vi "LightFieldParams.vi"(5 "On CCD Accumulations":i32=3 min=0 step=1, 7 "Number of Frames":i32=500 min=0 step=1, 8 "error in":errorcluster, 9 "BIN":u16(ring) items=["1x1", "2x2", "4x4"], 10 "MODE":u16(ring) items=["Normal", "DIF"], 11 "LightField Automation in":refnum<class "LightField Automation.lvclass">) -> (0 "error out":errorcluster, 3 "LightField Automation out":refnum<class "LightField Automation.lvclass">)   [LabVIEW 2018]
uses:
  <userlib>/LightField Add-in and Automation SDK/Samples/LabVIEW Automation/lightfield-automation-labview/LightField Automation.lvclass
  C:/Program Files/Princeton Instruments/LightField/PrincetonInstruments.LightFieldAddInSupportServices.dll
  Program Files/Princeton Instruments/LightField/PrincetonInstruments.LightFieldAddInSupportServices.dll
  C:/Program Files/Princeton Instruments/LightField/AddInViews/PrincetonInstruments.LightFieldViewV3.dll
  Program Files/Princeton Instruments/LightField/AddInViews/PrincetonInstruments.LightFieldViewV3.dll
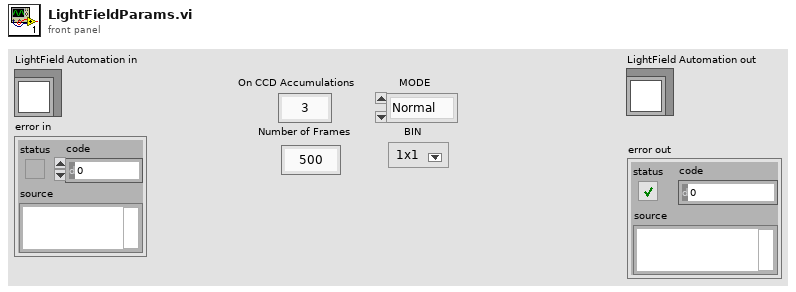
[diagram p1: front panel]
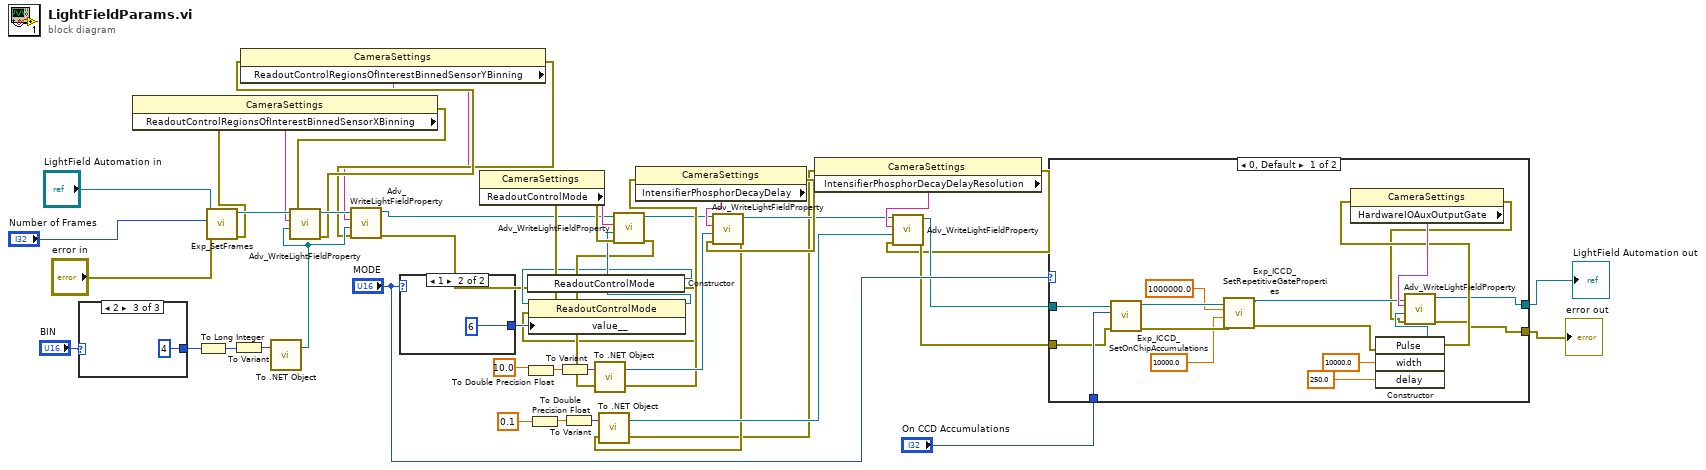
[diagram p0: block diagram]
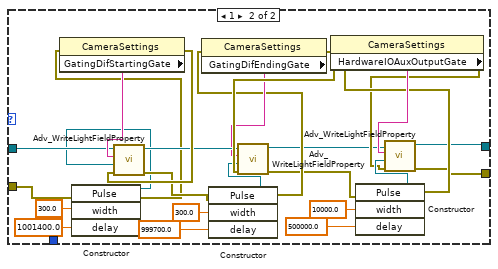
[diagram p2: hidden frame]
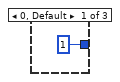
[diagram p3: hidden frame]
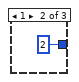
[diagram p4: hidden frame]
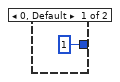
[diagram p5: hidden frame]
diagram:
  n1 = case shown="2" "BIN" {
    tunnel: [1 2 4] -> w19
    frame 0, Default {
    }
    frame 1 {
    }
    frame 2 {
    }
  }
  n2 = To Long Integer(number=w19) -> (32bit integer=w18:i32)
  n3 = call <userlib>:"Exp_SetFrames.vi"("error in (no error)"="error in", "Number of Frames"="Number of Frames", "LightField Automation in"="LightField Automation in") -> ("error out"=w30:errorcluster, "LightField Automation out"=w46:refnum<class "LightField Automation.lvclass">)  [unwired: 7 in]
  n4 = property class="CameraSettings"(error in=w30) -> (error out=w29:errorcluster, "ReadoutControlRegionsOfInterestBinnedSensorXBinning"=w28:string)  [unwired: 1 in, 1 out]
  n5 = To Variant(anything=w18) -> (Variant=w27:variant)
  n6 = call <vilib>:"To .NET Object.vi"("anything"=w27) -> (".NET object"=w26:refnum<k24>)  [unwired: 1 in, 1 out]
  n7 = call <userlib>:"Adv_WriteLightFieldProperty.vi"("error in (no error)"=w29, "value"=w26, "setting"=w28, "LightField Automation in"=w46) -> ("error out"=w25:errorcluster, "LightField Automation out"=w33:refnum<class "LightField Automation.lvclass">)  [unwired: 6 in]
  n8 = property class="CameraSettings"(error in=w25) -> (error out=w24:errorcluster, "ReadoutControlRegionsOfInterestBinnedSensorYBinning"=w23:string)  [unwired: 1 in, 1 out]
  n9 = call <userlib>:"Adv_WriteLightFieldProperty.vi"("error in (no error)"=w24, "value"=w26, "setting"=w23, "LightField Automation in"=w33) -> ("error out"=w21:errorcluster, "LightField Automation out"=w32:refnum<class "LightField Automation.lvclass">)  [unwired: 6 in]
  n10 = case shown="1" "MODE" {
    tunnel: [1 ("value__") 6 ("value__")] -> w43
    frame 0, Default {
    }
    frame 1 {
    }
  }
  n11 = To Double Precision Float(number=10.0) -> (double precision float=w17:dbl)
  n12 = constructor class="ReadoutControlMode"(error in=w21) -> (reference out=w22:refnum<k24>, error out=w20:errorcluster)  [unwired: 2 in, 1 out]
  n13 = property class="ReadoutControlMode"(reference=w22, error in=w20, "value__"=w43) -> (reference out=w42:refnum<k24>, error out=w41:errorcluster)
  n14 = property class="CameraSettings"(error in=w41) -> (error out=w44:errorcluster, "ReadoutControlMode"=w45:string)  [unwired: 1 in, 1 out]
  n15 = To Double Precision Float(number=0.1) -> (double precision float=w11:dbl)
  n16 = To Variant(anything=w17) -> (Variant=w39:variant)
  n17 = To Variant(anything=w11) -> (Variant=w12:variant)
  n18 = call <userlib>:"Adv_WriteLightFieldProperty.vi"("error in (no error)"=w44, "value"=w42, "setting"=w45, "LightField Automation in"=w32) -> ("error out"=w38:errorcluster, "LightField Automation out"=w34:refnum<class "LightField Automation.lvclass">)  [unwired: 6 in]
  n19 = call <vilib>:"To .NET Object.vi"("error in (no error)"=w38, "anything"=w39) -> ("error out"=w36:errorcluster, ".NET object"=w37:refnum<k24>)
  n20 = property class="CameraSettings"(error in=w36) -> (error out=w35:errorcluster, "IntensifierPhosphorDecayDelay"=w40:string)  [unwired: 1 in, 1 out]
  n21 = call <userlib>:"Adv_WriteLightFieldProperty.vi"("error in (no error)"=w35, "value"=w37, "setting"=w40, "LightField Automation in"=w34) -> ("error out"=w5:errorcluster, "LightField Automation out"=w8:refnum<class "LightField Automation.lvclass">)  [unwired: 6 in]
  n22 = call <vilib>:"To .NET Object.vi"("error in (no error)"=w5, "anything"=w12) -> ("error out"=w4:errorcluster, ".NET object"=w10:refnum<k24>)
  n23 = property class="CameraSettings"(error in=w4) -> (error out=w3:errorcluster, "IntensifierPhosphorDecayDelayResolution"=w9:string)  [unwired: 1 in, 1 out]
  n24 = call <userlib>:"Adv_WriteLightFieldProperty.vi"("error in (no error)"=w3, "value"=w10, "setting"=w9, "LightField Automation in"=w8) -> ("error out"=w6:errorcluster, "LightField Automation out"=w7:refnum<class "LightField Automation.lvclass">)  [unwired: 6 in]
  n25 = case shown="0, Default" "MODE" {
    tunnel: "On CCD Accumulations" -> [w71 _]
    tunnel: w6 -> [w70 w87]
    tunnel: w7 -> [w69 w96]
    tunnel: [w59 w74] -> w13
    tunnel: [w58 w73] -> w14
    frame 0, Default {
      n26 = call <userlib>:"Exp_ICCD_SetOnChipAccumulations.vi"("error in (no error)"=w70, "On Chip Accumulations"=w71, "LightField Automation in"=w69) -> ("error out"=w68:errorcluster, "LightField Automation out"=w67:refnum<class "LightField Automation.lvclass">)  [unwired: 7 in]
      n27 = call <userlib>:"Exp_ICCD_SetRepetitiveGateProperties.vi"("error in (no error)"=w68, "Repetitive Gate Width (ns)"=10000.0, "Repetitive Gate Delay (ns)"=1000000.0, "LightField Automation in"=w67) -> ("error out"=w60:errorcluster, "LightField Automation out"=w61:refnum<class "LightField Automation.lvclass">)  [unwired: 6 in]
      n28 = constructor class="Pulse"(error in=w60, "width"=10000.0 ("delay"), "delay"=250.0 ("width")) -> (reference out=w62:refnum<k24>, error out=w63:errorcluster)  [unwired: 2 in, 3 out]
      n29 = property class="CameraSettings"(error in=w63) -> (error out=w57:errorcluster, "HardwareIOAuxOutputGate"=w64:string)  [unwired: 1 in, 1 out]
      n30 = call <userlib>:"Adv_WriteLightFieldProperty.vi"("error in (no error)"=w57, "value"=w62, "setting"=w64, "LightField Automation in"=w61) -> ("error out"=w59:errorcluster, "LightField Automation out"=w58:refnum<class "LightField Automation.lvclass">)  [unwired: 6 in]
    }
    frame 1 {
      n31 = constructor class="Pulse"(error in=w87, "width"=300.0, "delay"=1001400.0) -> (reference out=w88:refnum<k24>, error out=w86:errorcluster)  [unwired: 2 in, 3 out]
      n32 = property class="CameraSettings"(error in=w86) -> (error out=w95:errorcluster, "GatingDifStartingGate"=w97:string)  [unwired: 1 in, 1 out]
      n33 = call <userlib>:"Adv_WriteLightFieldProperty.vi"("error in (no error)"=w95, "value"=w88, "setting"=w97, "LightField Automation in"=w96) -> ("error out"=w91:errorcluster, "LightField Automation out"=w93:refnum<class "LightField Automation.lvclass">)  [unwired: 6 in]
      n34 = constructor class="Pulse"(error in=w91, "width"=300.0, "delay"=999700.0) -> (reference out=w89:refnum<k24>, error out=w90:errorcluster)  [unwired: 2 in, 3 out]
      n35 = property class="CameraSettings"(error in=w90) -> (error out=w94:errorcluster, "GatingDifEndingGate"=w92:string)  [unwired: 1 in, 1 out]
      n36 = call <userlib>:"Adv_WriteLightFieldProperty.vi"("error in (no error)"=w94, "value"=w89, "setting"=w92, "LightField Automation in"=w93) -> ("error out"=w75:errorcluster, "LightField Automation out"=w72:refnum<class "LightField Automation.lvclass">)  [unwired: 6 in]
      n37 = constructor class="Pulse"(error in=w75, "width"=10000.0, "delay"=500000.0) -> (reference out=w79:refnum<k24>, error out=w80:errorcluster)  [unwired: 2 in, 3 out]
      n38 = property class="CameraSettings"(error in=w80) -> (error out=w76:errorcluster, "HardwareIOAuxOutputGate"=w81:string)  [unwired: 1 in, 1 out]
      n39 = call <userlib>:"Adv_WriteLightFieldProperty.vi"("error in (no error)"=w76, "value"=w79, "setting"=w81, "LightField Automation in"=w72) -> ("error out"=w74:errorcluster, "LightField Automation out"=w73:refnum<class "LightField Automation.lvclass">)  [unwired: 6 in]
    }
  }
  "error out" <- w13
  "LightField Automation out" <- w14
